vi "HistoDataToChannelFormat.vi"(8 "error in":errorcluster, 11 "Histo Bins":i32[](array[numeric])) -> (0 "error out":errorcluster, 3 "Channel Data":dbl[](array[numeric]))   [LabVIEW 2012, in "Histogram Custom Device.lvlib"]
uses:
  Histogram Custom Device.lvlib
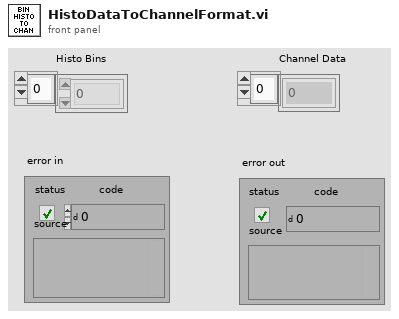
[diagram p1: front panel]
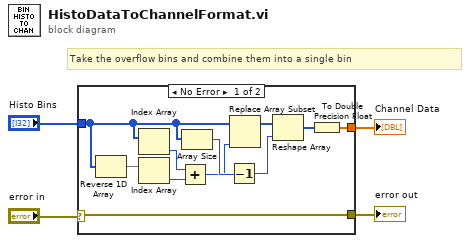
[diagram p0: block diagram]
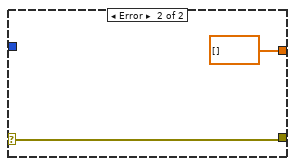
[diagram p2: hidden frame]
diagram:
  # "Take the overflow bins and combine them into a single bin"
  n1 = case shown="No Error" "error in" {
    selector: "error in" -> [w5 w17]
    tunnel: "Histo Bins" -> [w8 _]
    tunnel: [w6 dbl[] []] -> w3
    tunnel: [w5 w17] -> w1
    frame No Error {
      n2 = Reverse 1D Array(array=w8) -> (reversed array=w9:i32[])
      n3 = Index Array(array=w8) -> (element=w10:i32)  [unwired: 1 in]
      n4 = Index Array(array=w9) -> (element=w11:i32)  [unwired: 1 in]
      n5 = Add(x=w10, y=w11) -> (x+y=w12:i32)
      n6 = Array Size(array=w8) -> (size(s)=w14:i32)
      n7 = Decrement(x=w14) -> (x-1=w15:i32)
      n8 = Replace Array Subset(array=w8, new element=w12) -> (w13:i32[])  [unwired: 1 in]
      n9 = Reshape Array(w13, w15) -> (w7:i32[])
      n10 = To Double Precision Float(number=w7) -> (double precision float=w6:dbl[])
    }
    frame Error {
    }
  }
  "Channel Data" <- w3
  "error out" <- w1
